vi "Core-EnQueueMultiElements.vi"(8 "ErrorIn":errorcluster, 10 "CmdArray":cluster{"State":string, "Data":variant}[](array[cluster]), 11 "QRefIn":refnum<queue>) -> (0 "ErrorOut":errorcluster)   [LabVIEW 2021]
doc: "Enqueue Multi Elements\n- Enqueue all elements in arrary to queue.\n\nNotes:\n- N/A"
panel:
  # "Inputs"
  # "Outputs"
  # ":: Modularized Parallism Templete ::\n- EnQueue MultiElements -\nby: Techie <HighTechYoung@yahoo.com>\nCopyright (C) 2010, Vision Technologies All Rights Reserved"
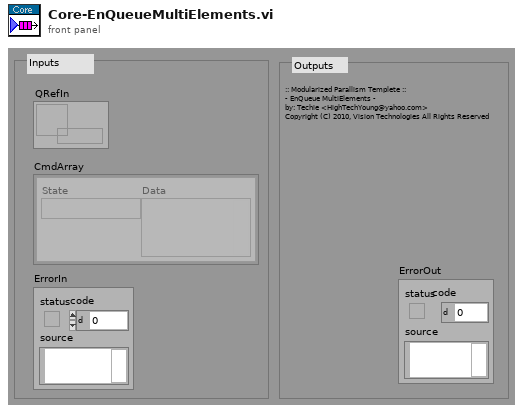
[diagram p1: front panel]
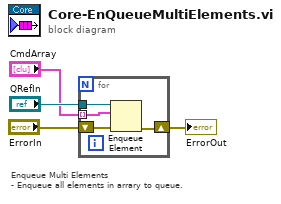
[diagram p0: block diagram]
diagram:
  # "Enqueue Multi Elements\n- Enqueue all elements in arrary to queue."
  n1 = for {
    shift-right: [w7] -> w3
    shift-left: "ErrorIn" -> [w8]
    tunnel: "QRefIn" -> [w6]
    tunnel: "CmdArray" -> [w5] mode=indexing
    n2 = Enqueue Element(queue=w6, element=w5, error in (no error)=w8) -> (error out=w7:errorcluster)  [unwired: 3 out]
  }
  "ErrorOut" <- w3
